vi "Elevator Height Selector.vi"(6 "M down":bool, 7 "M up":bool, 9 "Top":bool, 10 "Tote on Tote":bool, 11 "Bottom":bool) -> (3 "Numeric":dbl)   [LabVIEW 2014]
uses:
  Robot Global Data.vi
panel:
  # ".22\n.55\n.95\n.01"
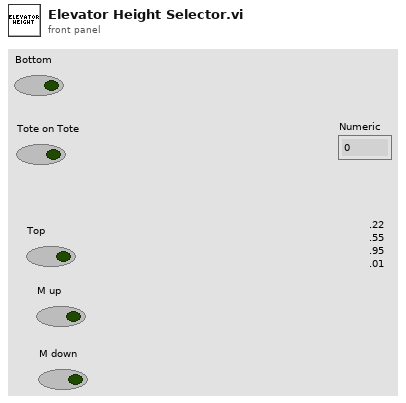
[diagram p1: front panel]
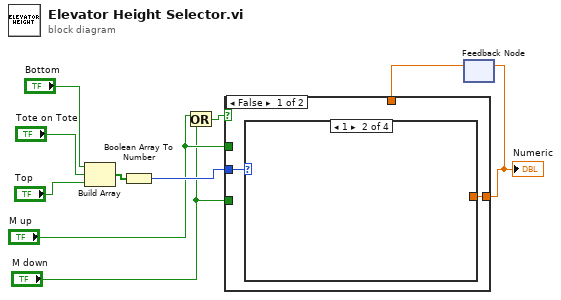
[diagram p0: block diagram]
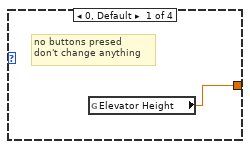
[diagram p2: hidden frame]
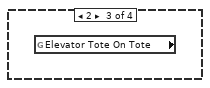
[diagram p3: hidden frame]
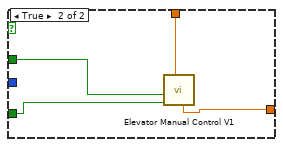
[diagram p5: hidden frame]
diagram:
  n1 = Build Array("Bottom", "Tote on Tote", "Top") -> (w10:bool[])
  n2 = Boolean Array To Number(Boolean array=w10) -> (number=w7:u32)
  n3 = Or(x="M up", y="M down") -> (x .or. y?=w6:bool)
  n4 = feedback #1() -> (w2:dbl)  [unwired: 1 in]
  n5 = case shown="False" w6 {
    tunnel: [w11 w17] -> w1
    tunnel: w7 -> [w12 _]
    tunnel: "M up" -> [_ w16]
    tunnel: "M down" -> [_ w15]
    tunnel: w2 -> [_ w14]
    frame False {
      n6 = case shown="1" w12 {
        tunnel: [w13 _ _ _] -> w11
        frame 0, Default {
          # "no buttons presed\ndon't change anything"
          n7 = global read "Robot Global Data.vi" "Elevator Height"() -> (w13:dbl)
        }
        frame 1 {
        }
        frame 2 {
          n8 = global read "Robot Global Data.vi" "Elevator Tote On Tote"() -> ()  [unwired: 1 out]
        }
        frame 4 {
        }
      }
    }
    frame True {
      n9 = call "Elevator Manual Control V1.vi"("Input"=w14, "Down"=w15, "Up"=w16) -> ("Output"=w17:dbl)  [unwired: 8 in]
    }
  }
  "Numeric" <- w1
  n10 = feedback-in #1(w1) -> ()
